vi "QCP_Get_STR_Array.vi"(0 "Data Value Reference in":T1, 1 "String":string, 3 "error in (no error)":errorcluster) -> (7 "Data Value Reference Out":T1, 8 "Array":string[](array[string]), 10 "Error Out":errorcluster)   [LabVIEW 2016]
uses:
  <userlib>/836-Libraries/System/QCP_Support_Code/QCP_Data_Block.ctl
  <userlib>/836-Libraries/System/QCP_Support_Code/QCP_Get_STR.vi
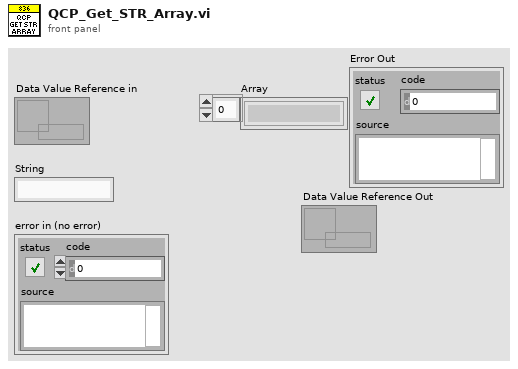
[diagram p1: front panel]
types:
  T1 = typedef "QCP_Data_Block.ctl" = refnum<data-value>
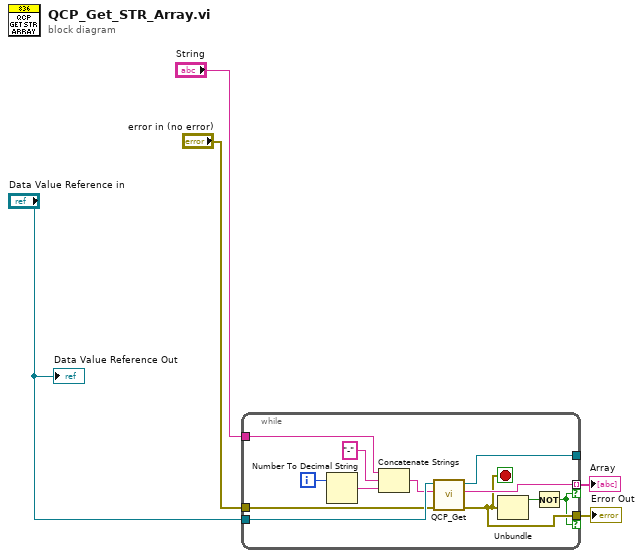
[diagram p0: block diagram]
diagram:
  n1 = while {
    tunnel: "String" -> [w17]
    tunnel: "Data Value Reference in" -> [w16]
    tunnel: [w12] -> _
    tunnel: "error in (no error)" -> [w11]
    tunnel: [w8] -> w5 mode=indexing if=w6
    tunnel: [w7] -> w1 if=w6
    i -> [w10]
    stop <- w7 stop-if-true
    n2 = Number To Decimal String(number=w10) -> (decimal integer string=w14:string)  [unwired: 1 in]
    n3 = Concatenate Strings(w17, "-" ("string"), w14) -> (w13:string)
    n4 = call-poly <userlib>:"QCP_Get.vi"("QCP Data Block In"=w16, "QCP Name"=w13, "Error In"=w11) -> ("QCP Data Block Out"=w12:T1, "Value Out"=w8:string, "Error Out"=w7:errorcluster)  [unwired: 5 in]
    n5 = Unbundle(w7) -> ("status"=w9:bool)  [unwired: 2 out]
    n6 = Not(x=w9) -> (.not. x?=w6:bool)
  }
  "Array" <- w5
  "Error Out" <- w1
  "Data Value Reference Out" <- "Data Value Reference in"
